vi "Set ILog Data.vi"(10 "ILog Data":refnum<class "ILog Data.lvclass">, 11 "Action Point in":refnum<class "Action Point.lvclass">) -> (3 "Action Point out":refnum<class "Action Point.lvclass">)   [LabVIEW 2025, in "Action Point.lvclass"]
uses:
  Action Point.lvclass
  Interfaces/ILog Data/ILog Data.lvclass
  Action Point.lvclass/Action Point.ctl
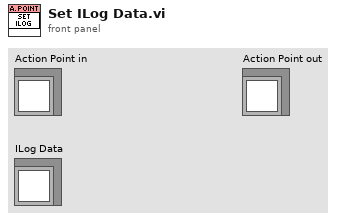
[diagram p1: front panel]
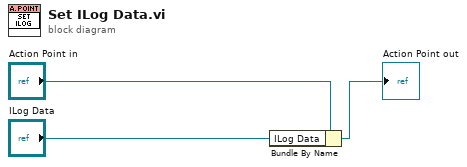
[diagram p0: block diagram]
diagram:
  n1 = Bundle By Name(cluster="Action Point in", "ILog Data"="ILog Data") -> (→"Action Point out":refnum<class "Action Point.lvclass">)
